vi "monochromatorConnect.vi"(8 "error in":errorcluster, 10 "product_id":i32 format="%x", 11 "vendor_id":i32 format="%x") -> (0 "error out":errorcluster, 3 "monochromator":refnum<k24>)   [LabVIEW 2009]
doc: "This VI is responsible for connecting to Oriel/Newport Monochromator. \n\nIt will return monochromator .net reference if connection is sucessful, otherwise it will throw error 90101 - \"Error Initializing Monochromator and return empty .net reference"
uses:
  C:/Users/anderson.chen/Desktop/Software Development/Cornerstone Series API (LV9)/Cornerstone DLL/Cornerstone.dll
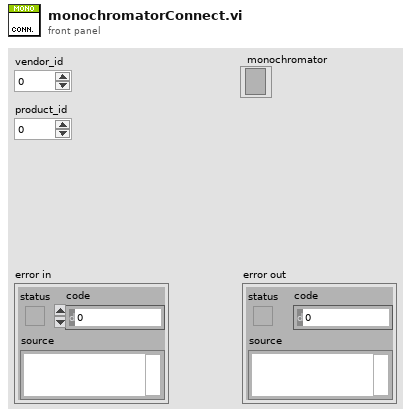
[diagram p1: front panel]
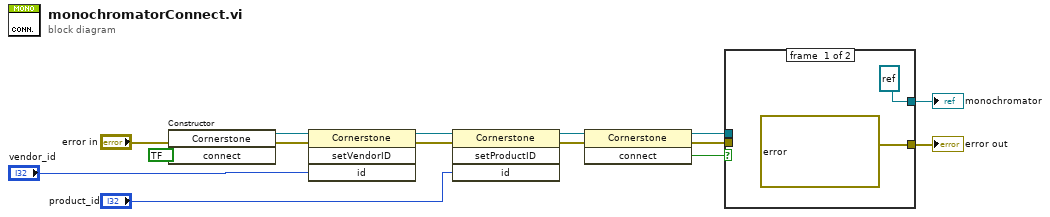
[diagram p0: block diagram]
diagram:
  n1 = constructor class="Cornerstone"(error in="error in", "connect"=bool ?) -> (reference out=w14:refnum<k24>, error out=w6:errorcluster)  [unwired: 2 in, 2 out]
  n2 = invoke class="Cornerstone" method="setVendorID"(reference=w14, error in=w6, "id"="vendor_id") -> (reference out=w7:refnum<k24>, error out=w3:errorcluster)  [unwired: 1 in, 2 out]
  n3 = invoke class="Cornerstone" method="setProductID"(reference=w7, error in=w3, "id"="product_id") -> (reference out=w4:refnum<k24>, error out=w2:errorcluster)  [unwired: 1 in, 2 out]
  n4 = invoke class="Cornerstone" method="connect"(reference=w4, error in=w2) -> (reference out=w12:refnum<k24>, error out=w11:errorcluster, "connect"=w13:bool)  [unwired: 1 in]
  n5 = case shown="True" w13 {
    tunnel: w12 -> [_ w19]
    tunnel: [refnum<k24> ? ("new reference") w19] -> w9
    tunnel: w11 -> [_ w18]
    tunnel: [errorcluster ? ("error out") w18] -> w8
    frame #0 {
    }
    frame #1 {
    }
  }
  "monochromator" <- w9
  "error out" <- w8
